vi "TaskManager.vi"() -> ()   [LabVIEW 2020]
panel:
  out "min value":dbl caption="min" format="%0.1f %"
  out "max value":dbl caption="max" format="%0.1f %"
  out "CPU Load, %":dbl(graph)
  out "Memory Usage":u32(graph)
  in  "Empty":bool
  in  "Process list":i32(listbox)=-1
  in  "stop":bool=TRUE
  # "Current"
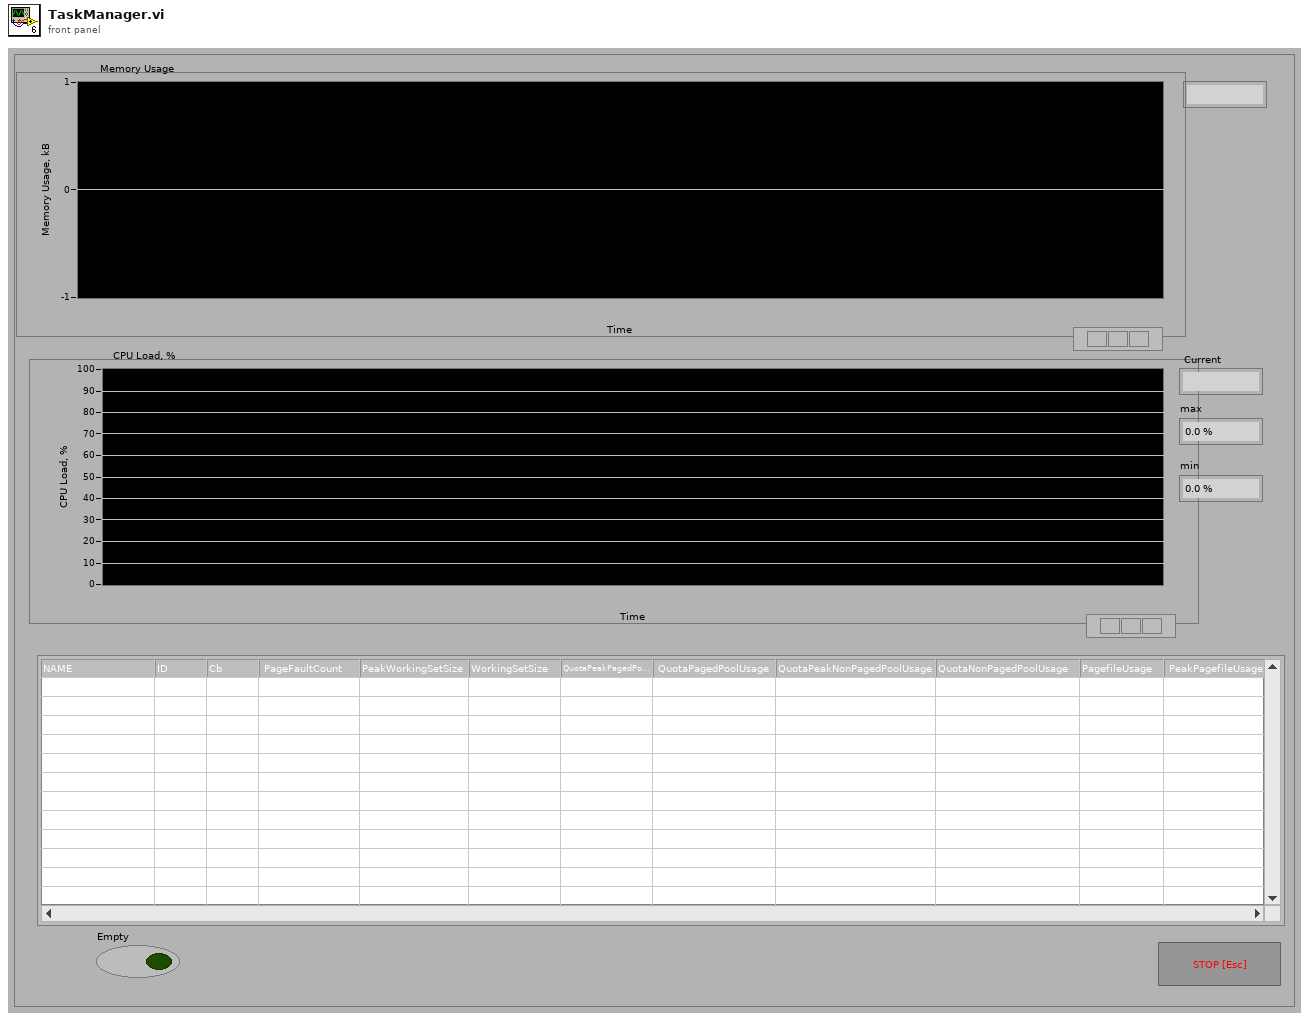
[diagram p1: front panel]
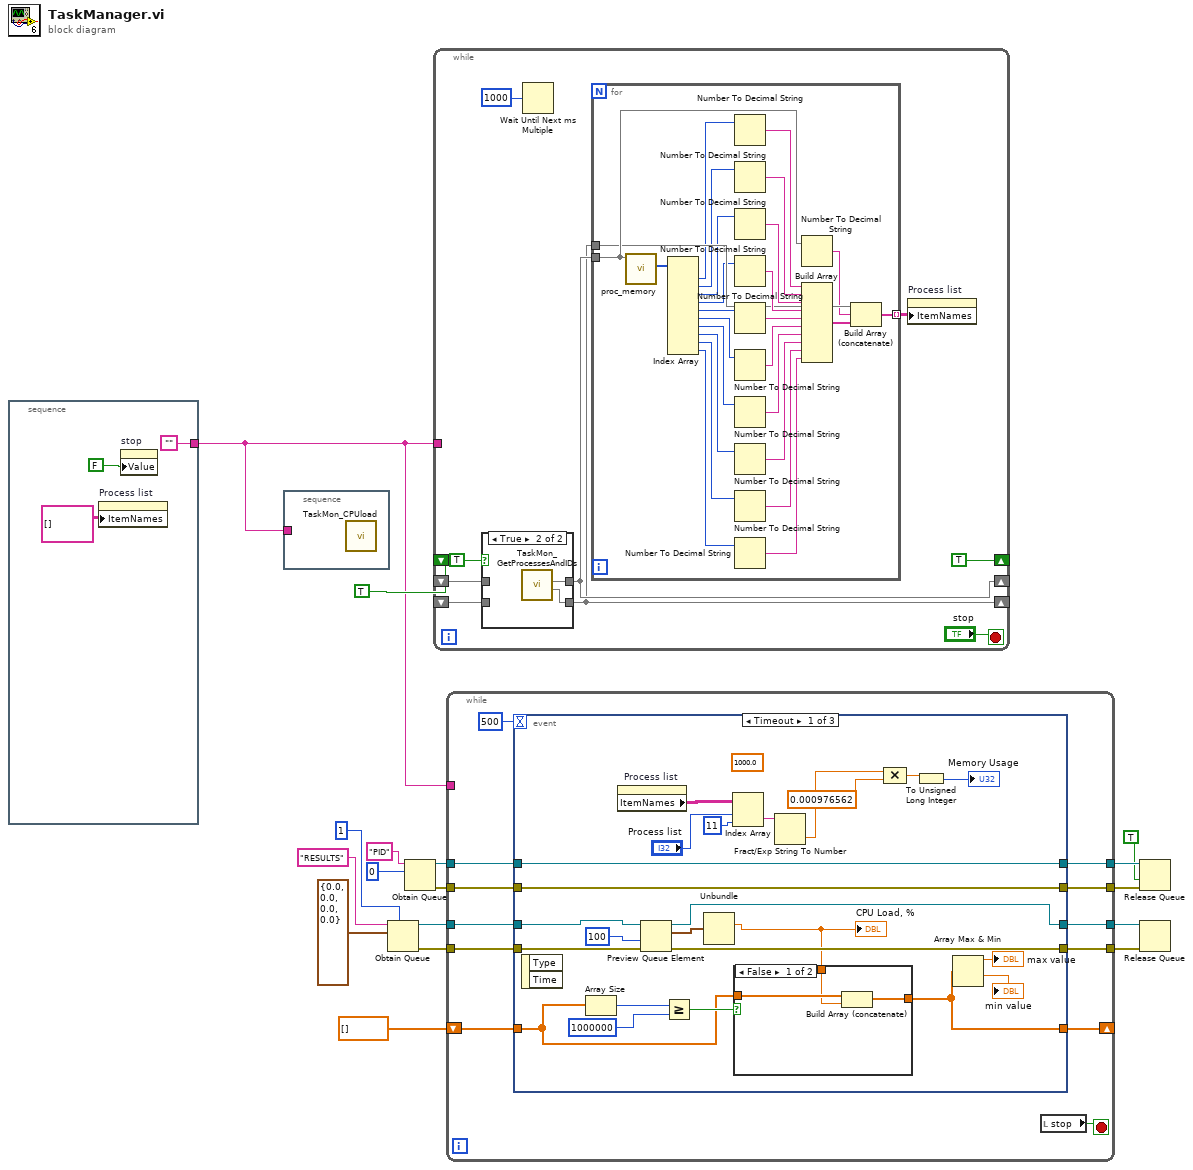
[diagram p0: block diagram]
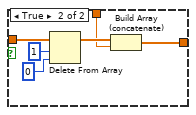
[diagram p2: hidden frame]
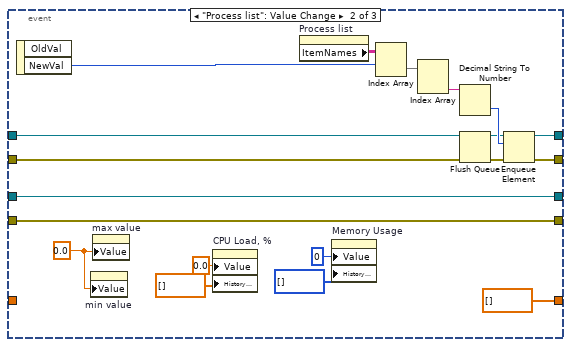
[diagram p3: hidden frame]
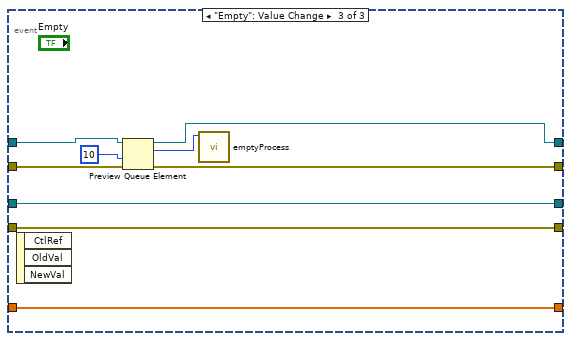
[diagram p4: hidden frame]
diagram:
  n1 = stacked-sequence {
    tunnel: [""] -> w1
    frame #0 {
      n2 = property on="Process list" class="MCListbox (strict)"("ItemNames"=string[][] [] ("Item Names")) -> ()  [unwired: 2 in, 2 out]
      n3 = property on="stop" class="Bool (strict)"("Value"=FALSE ("stop")) -> ()  [unwired: 2 in, 2 out]
    }
  }
  n4 = stacked-sequence {
    tunnel: w1 -> [_]
    frame #0 {
      n5 = call "TaskMon_CPUload.vi"() -> ()  [unwired: 10 in, 2 out]
    }
  }
  n6 = Obtain Queue(max queue size (-1, unlimited)=1, name (unnamed)="RESULTS", element data type=cluster{dbl, dbl, dbl, dbl} {0.0, 0.0, 0.0, 0.0}) -> (queue out=w9:refnum<queue>, error out=w8:errorcluster)  [unwired: 2 in, 1 out]
  n7 = Obtain Queue(name (unnamed)="PID", element data type=0) -> (queue out=w14:refnum<queue>, error out=w13:errorcluster)  [unwired: 3 in, 1 out]
  n8 = while {
    shift-right: [w26] -> _
    shift-left: _ -> [w25]
    shift-right: [w24] -> _
    shift-left: _ -> [w23]
    shift-right: [TRUE] -> _
    shift-left: TRUE -> [_]
    tunnel: w1 -> [_]
    stop <- "stop" stop-if-true
    n9 = case shown="True" TRUE {
      tunnel: [w31 w33] -> w26
      tunnel: [w30 w32] -> w24
      tunnel: w25 -> [w31 _]
      tunnel: w23 -> [w30 _]
      frame False {
      }
      frame True {
        n10 = call "TaskMon_GetProcessesAndIDs.vi"() -> (1:w32, 2:w33)  [unwired: 1 in, 9 out]
      }
    }
    n11 = Wait Until Next ms Multiple(millisecond multiple=u32 1000) -> ()  [unwired: 1 out]
    n12 = for {
      tunnel: w26 -> [w50]
      tunnel: w24 -> [w49]
      tunnel: [w46] -> w27 mode=indexing
      n13 = call "proc_memory.vi"("id"=w50) -> ("info 2"=w45:u32[])  [unwired: 10 out]
      n14 = Index Array(array=w45) -> (element #1=w44:u32, element #2=w43:u32, element #3=w42:u32, element #4=w41:u32, element #5=w40:u32, element #6=w39:u32, element #7=w38:u32, element #8=w37:u32, element #9=w36:u32, element #10=w35:u32)  [unwired: 10 in]
      n15 = Number To Decimal String(number=w44) -> (decimal integer string=w59:string)  [unwired: 1 out]
      n16 = Number To Decimal String(number=w43) -> (decimal integer string=w58:string)  [unwired: 1 out]
      n17 = Number To Decimal String(number=w42) -> (decimal integer string=w57:string)  [unwired: 1 out]
      n18 = Number To Decimal String(number=w41) -> (decimal integer string=w56:string)  [unwired: 1 out]
      n19 = Number To Decimal String(number=w40) -> (decimal integer string=w55:string)  [unwired: 1 out]
      n20 = Number To Decimal String(number=w39) -> (decimal integer string=w54:string)  [unwired: 1 out]
      n21 = Number To Decimal String(number=w38) -> (decimal integer string=w53:string)  [unwired: 1 out]
      n22 = Number To Decimal String(number=w37) -> (decimal integer string=w52:string)  [unwired: 1 out]
      n23 = Number To Decimal String(number=w36) -> (decimal integer string=w51:string)  [unwired: 1 out]
      n24 = Number To Decimal String(number=w35) -> (decimal integer string=w34:string)  [unwired: 1 out]
      n25 = Number To Decimal String(number=w50) -> (decimal integer string=w48:string)  [unwired: 1 out]
      n26 = Build Array(w59, w58, w57, w56, w55, w54, w53, w52, w51, w34) -> (w47:string[])
      n27 = Build Array (concatenate)(w49, w48, w47) -> (w46:string[])
    }
    n28 = property on="Process list" class="MCListbox (strict)"("ItemNames"=w27) -> ()  [unwired: 2 in, 2 out]
  }
  n29 = while {
    tunnel: w14 -> [w71]
    tunnel: w13 -> [w70]
    tunnel: w9 -> [w69]
    tunnel: w8 -> [w68]
    tunnel: [w65] -> w6
    tunnel: [w64] -> w7
    tunnel: [w63] -> w3
    tunnel: [w62] -> w4
    tunnel: w1 -> [_]
    shift-right: [w60] -> _
    shift-left: dbl[] [] -> [w61]
    stop <- w67 stop-if-true
    n30 = event shown="[0] Timeout" {
      selector: _ -> [_ _ _]
      dyn-events: _ -> [_ _ _]
      timeout: 500 -> [_ _ _]
      tunnel: w71 -> [w84 w114 w131]
      tunnel: w70 -> [w83 w113 w132]
      tunnel: w69 -> [w95 w116 w126]
      tunnel: w68 -> [w94 w115 w125]
      tunnel: [w84 w118 w128] -> w65
      tunnel: [w83 w117 w127] -> w64
      tunnel: [w82 w116 w126] -> w63
      tunnel: [w81 w115 w125] -> w62
      tunnel: w61 -> [w76 _ w124]
      tunnel: [w74 dbl[] [] w124] -> w60
      event Timeout {
        (unwired) 1000.0 ("y")
        n31 = event-data() -> ()  [unwired: 1 in, 2 out]
        n32 = Array Size(array=w76) -> (size(s)=w79:i32)
        n33 = property on="Process list" class="MCListbox (strict)"() -> ("ItemNames"=w91:string[][])  [unwired: 2 in, 2 out]
        n34 = Preview Queue Element(queue=w95, timeout in ms (-1)=100, error in (no error)=w94) -> (queue out=w82:refnum<queue>, element=w92:cluster{dbl, dbl, dbl, dbl}, error out=w81:errorcluster)  [unwired: 1 out]
        n35 = Greater Or Equal?(x=w79, y=1000000) -> (x >= y?=w77:bool)
        n36 = Unbundle(w92) -> (w75:dbl)  [unwired: 3 out]
        "CPU Load, %" <- w75
        n37 = Index Array(array=w91, index (row)="Process list", index (col)=11 ("disabled index (col)")) -> (element=w88:string)
        n38 = case shown="False" w77 {
          tunnel: w76 -> [w98 w104]
          tunnel: w75 -> [w97 w100]
          tunnel: [w96 w99] -> w74
          frame False {
            n39 = Build Array (concatenate)(w98, w97) -> (w96:dbl[])
          }
          frame True {
            n40 = Delete From Array(array=w104, length=1, index=0) -> (array with subset deleted=w101:dbl[])  [unwired: 1 out]
            n41 = Build Array (concatenate)(w101, w100) -> (w99:dbl[])
          }
        }
        n42 = Fract/Exp String To Number(string=w88) -> (number=w87:dbl)  [unwired: 3 in, 1 out]
        n43 = Compound Arithmetic op=MULTIPLY(w87, 0.000976562 ("value")) -> (w85:dbl)
        n44 = To Unsigned Long Integer(number=w85) -> (unsigned 32bit integer=→"Memory Usage":u32)
        n45 = Array Max & Min(array=w74) -> (max value=→"max value":dbl, min value=→"min value":dbl)  [unwired: 2 out]
      }
      event "Process list": Value Change {
        w110 = 0.0 ("CPU Load, %")
        n46 = event-data() -> ("NewVal"=w122:i32)  [unwired: 1 in, 1 out]
        n47 = property on="min value" class="DigNum (strict)"("Value"=w110) -> ()  [unwired: 2 in, 2 out]
        n48 = property on="max value" class="DigNum (strict)"("Value"=w110) -> ()  [unwired: 2 in, 2 out]
        n49 = property on="CPU Load, %" class="WFChart (strict)"("Value"=0.0 ("CPU Load, %"), "History Data"=dbl[] []) -> ()  [unwired: 2 in, 2 out]
        n50 = property on="Process list" class="MCListbox (strict)"() -> ("ItemNames"=w123:string[][])  [unwired: 2 in, 2 out]
        n51 = property on="Memory Usage" class="WFChart (strict)"("Value"=0 ("Memory Usage"), "History Data"=i32[] []) -> ()  [unwired: 2 in, 2 out]
        n52 = Index Array(array=w123, index (row)=w122) -> (element=w121:string[])  [unwired: 1 in]
        n53 = Index Array(array=w121) -> (element #2=w120:string)  [unwired: 2 in, 1 out]
        n54 = Decimal String To Number(string=w120) -> (number=w119:i32)  [unwired: 2 in, 1 out]
        n55 = Flush Queue(queue=w114, error in (no error)=w113) -> (queue out=w112:refnum<queue>, error out=w111:errorcluster)  [unwired: 1 out]
        n56 = Enqueue Element(queue=w112, element=w119, error in (no error)=w111) -> (queue out=w118:refnum<queue>, error out=w117:errorcluster)  [unwired: 1 in, 1 out]
      }
      event "Empty": Value Change {
        n57 = event-data() -> ()  [unwired: 1 in, 3 out]
        n58 = Preview Queue Element(queue=w131, timeout in ms (-1)=10, error in (no error)=w132) -> (queue out=w128:refnum<queue>, element=w129:i32, error out=w127:errorcluster)  [unwired: 1 out]
        n59 = call "emptyProcess.vi"("ID"=w129) -> ()  [unwired: 1 in, 10 out]
      }
    }
    n60 = local read "stop"() -> (w67:bool)
  }
  n61 = Release Queue(queue=w6, force destroy? (F)=TRUE, error in (no error)=w7) -> ()  [unwired: 3 out]
  n62 = Release Queue(queue=w3, error in (no error)=w4) -> ()  [unwired: 1 in, 3 out]
